vi "Configure Power Measurement List TX Increment Mode.vi"(8 "error in (no error)":errorcluster, 9 "Mode (Index Repetition)":i32(ring) items=["Index Repetition", "List Entry"], 10 "Instance (1)":i32=1, 11 "VISA resource name":refnum<visa-resource-name>) -> (0 "error out":errorcluster, 3 "VISA resource name out":refnum<visa-resource-name>)   [LabVIEW 2020, in "Rohde&Schwarz CMXP GPRF.lvlib"]
doc: "Selects the repetition of the GPRF Meas<i>:Power trigger signal, generated by the power measurement for a repeated segment.\n\nAttribute:\nRSCMXPGPRF_ATTR_POWER_MEASUREMENT_LIST_TX_INCREMENT_MODE\n\nRemote-control command:\nCONFigure:GPRF:MEAS<i>:POWer:LIST:TXIMode"
uses:
  <instrlib>/Rohde&Schwarz CMXP GPRF/Rohde&Schwarz CMXP GPRF.lvlib
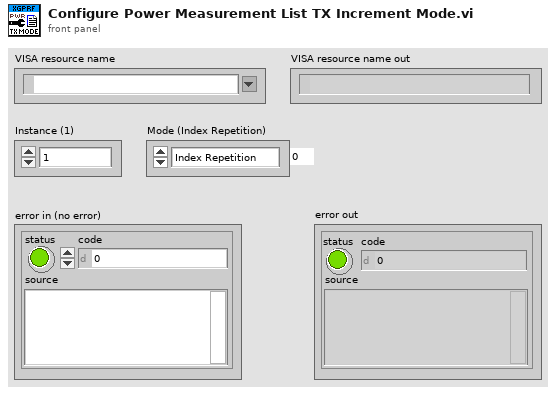
[diagram p1: front panel]
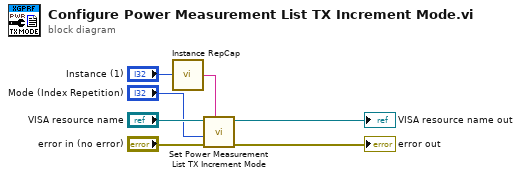
[diagram p0: block diagram]
diagram:
  n1 = call <instrlib>:"Instance RepCap.vi"("Instance in"="Instance (1)") -> ("Instance out"=w7:string)
  n2 = call "Set Power Measurement List TX Increment Mode"("Repeated Capabilities"=w7, "error in (no error)"="error in (no error)", "Power Measurement List TX Increment Mode (0 - Index Repetition)"="Mode (Index Repetition)", "instrument handle"="VISA resource name") -> ("error out"=→"error out":errorcluster, "instrument handle out"=→"VISA resource name out":refnum<visa-resource-name>)  [unwired: 6 in]
